vi "Read Registered Sinks Event Ref.vi"(8 "error in (no error)":errorcluster, 11 "Event Source in":refnum<class "Event Source.lvclass">) -> (0 "error out":errorcluster, 2 "Registerd Sinks Event Ref":T1, 3 "Event Source out":refnum<class "Event Source.lvclass">)   [LabVIEW 2016, in "Event Source.lvlib" / "Event Source.lvclass"]
uses:
  Event Source.lvclass
  Registered Sinks Event Ref.ctl
  Event Source.lvclass/Event Source.ctl
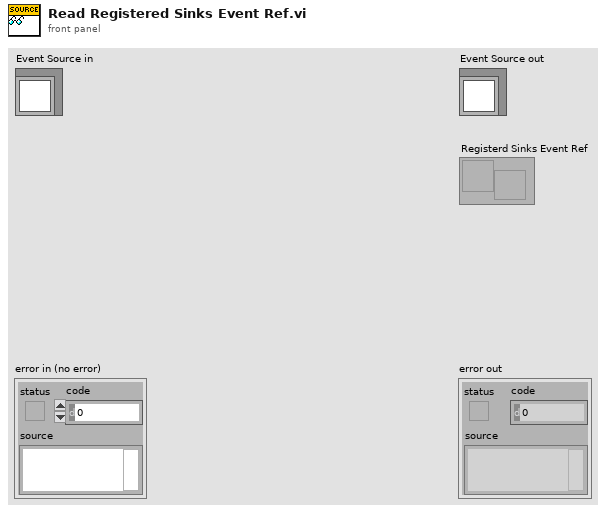
[diagram p1: front panel]
types:
  T1 = typedef "Event Source.lvlib/Event Source.lvclass/Registered Sinks Event Ref.ctl" = refnum<user-event>
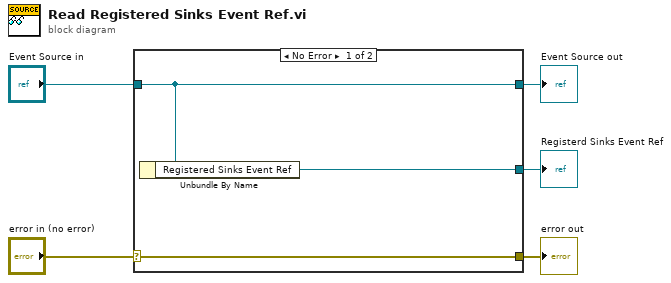
[diagram p0: block diagram]
diagram:
  n1 = case shown="No Error" "error in (no error)" {
    selector: "error in (no error)" -> [w8 w9]
    tunnel: [w8 w9] -> w4
    tunnel: [w7 w10] -> w2
    tunnel: "Event Source in" -> [w7 w10]
    tunnel: [w6 _] -> w1
    frame No Error {
      n2 = Unbundle By Name(w7) -> ("Registered Sinks Event Ref"=w6:T1)
    }
    frame Error {
    }
  }
  "error out" <- w4
  "Event Source out" <- w2
  "Registerd Sinks Event Ref" <- w1
